vi "Update_Grid_Resolution_SubVI.vi"(10 "X pixel":i32, 11 "Y pixel":i32) -> ()   [LabVIEW 2014]
uses:
  <userlib>/Nanonis Prog Interface V5/Scan/Grid/GridPatternSet.vi
  <userlib>/Nanonis Prog Interface V5/Nanonis Prog Interface.lvlib
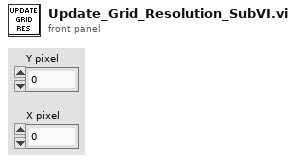
[diagram p1: front panel]
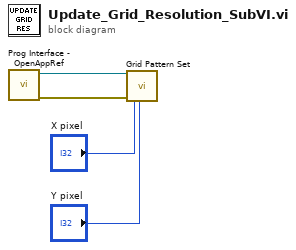
[diagram p0: block diagram]
diagram:
  n1 = call <userlib>:"Prog Interface - OpenAppRef.vi"() -> ("Error out"=w1:errorcluster, "Application reference"=w2:refnum<vi>)  [unwired: 6 in]
  n2 = call-poly <userlib>:"Grid Pattern Set.vi"("Application ref in"=w2, "error in (no error)"=w1, "Points X"="X pixel", "Points Y"="Y pixel") -> ()  [unwired: 14 in, 2 out]
